vi "Configure Bias Level.vi"(8 "error in (no error)":errorcluster, 9 "Channel List(\"\")":string, 10 "Bias (1: 0.001A)":i32(ring)=1 items=["0.0001", "0.001", "0.01"], 11 "VISA resource name":refnum<visa-resource-name>) -> (0 "error out":errorcluster, 3 "VISA resource name out":refnum<visa-resource-name>)   [LabVIEW 2016, in "Keithley DMM6500 DAQ6500 Series.lvlib"]
doc: "Selects the amount of current the instrument sources when it makes measurements."
uses:
  Keithley DMM6500 DAQ6500 Series.lvlib
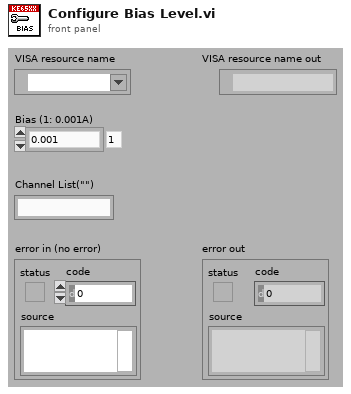
[diagram p1: front panel]
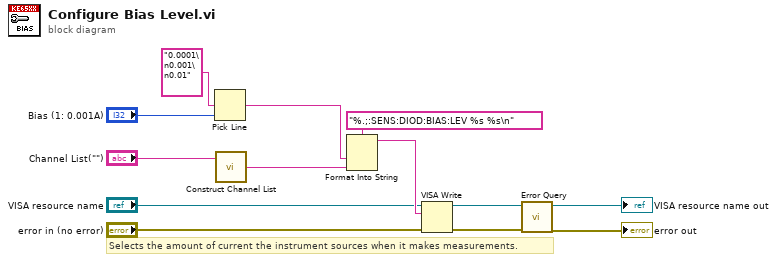
[diagram p0: block diagram]
diagram:
  # "Selects the amount of current the instrument sources when it makes measurements."
  n1 = Pick Line(multi-line string="0.0001\n0.001\n0.01", line index="Bias (1: 0.001A)") -> (output string=w1:string)  [unwired: 1 in]
  n2 = call "Construct Channel List.vi"("Channel List"="Channel List(\"\")") -> ("Channel List String"=w4:string)  [unwired: 2 in]
  n3 = Format Into String(format string="%.;:SENS:DIOD:BIAS:LEV %s %s\n", w1, w4) -> (resulting string=w12:string)  [unwired: 2 in, 1 out]
  n4 = VISA Write(VISA resource name="VISA resource name", write buffer=w12, error in (no error)="error in (no error)") -> (VISA resource name out=w9:refnum<visa-resource-name>, error out=w8:errorcluster)  [unwired: 1 out]
  n5 = call "Error Query.vi"("error in (no error)"=w8, "VISA resource name"=w9) -> ("error out"=→"error out":errorcluster, "VISA resource name out"=→"VISA resource name out":refnum<visa-resource-name>)  [unwired: 6 in, 2 out]
